vi "ChAndCoreXMLPaths.vi"(6 "Esis":string, 9 "Egi2":string, 10 "Core":string, 11 "Egi1":string) -> (1 "Egi1 Xml Path":path, 2 "Esis Xml Path":path, 3 "Egi2 Xml Path":path, 4 "Core Xml Path":path)   [LabVIEW 2023]
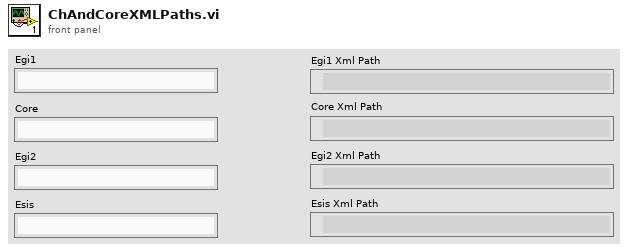
[diagram p1: front panel]
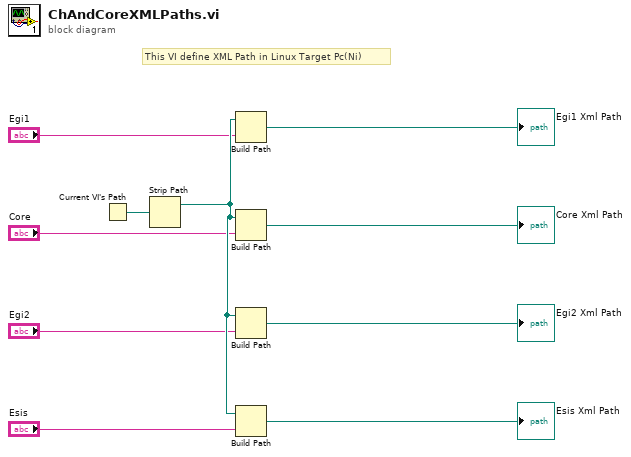
[diagram p0: block diagram]
diagram:
  # "This VI define XML Path in Linux Target Pc(Ni)"
  n1 = Current VI's Path() -> (path=w1:path)
  n2 = Strip Path(path=w1) -> (stripped path=w9:path)  [unwired: 1 out]
  n3 = Build Path(base path=w9, name or relative path="Egi1") -> (appended path=→"Egi1 Xml Path":path)
  n4 = Build Path(base path=w9, name or relative path="Core") -> (appended path=→"Core Xml Path":path)
  n5 = Build Path(base path=w9, name or relative path="Egi2") -> (appended path=→"Egi2 Xml Path":path)
  n6 = Build Path(base path=w9, name or relative path="Esis") -> (appended path=→"Esis Xml Path":path)
